vi "DetectDev.vi"(1 "IP.":string caption="IP地址") -> (0 "Fail":bool)   [LabVIEW 2012]
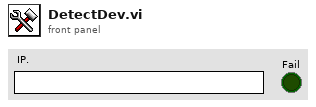
[diagram p1: front panel]
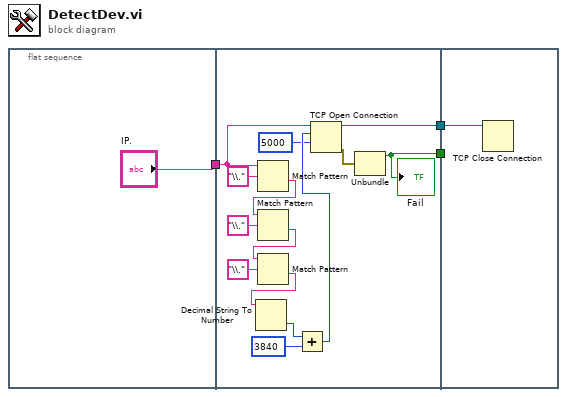
[diagram p0: block diagram]
diagram:
  n1 = flat-sequence {
    tunnel: ["IP."] -> w3
    tunnel: w3 -> [w13]
    tunnel: [w7] -> w2
    tunnel: [w6] -> w1
    tunnel: w2 -> [w19]
    tunnel: w1 -> [_]
    frame #0 {
    }
    frame #1 {
      n2 = Match Pattern(string=w13, regular expression="\\." ("正则表达式")) -> (after substring=w15:string)  [unwired: 1 in, 3 out]
      n3 = Match Pattern(string=w15, regular expression="\\." ("正则表达式")) -> (after substring=w14:string)  [unwired: 1 in, 3 out]
      n4 = Match Pattern(string=w14, regular expression="\\." ("正则表达式")) -> (after substring=w12:string)  [unwired: 1 in, 3 out]
      n5 = Decimal String To Number(string=w12) -> (number=w11:i32)  [unwired: 2 in, 1 out]
      n6 = Add(x=w11, y=3840) -> (x+y=w9:i32)
      n7 = TCP Open Connection(address=w13, remote port or service name=w9, timeout ms (60000)=5000 ("超时毫秒(60000)")) -> (connection ID=w7:refnum<k5>, error out=w8:errorcluster)  [unwired: 2 in]
      n8 = Unbundle(w8) -> ("status"=w6:bool)  [unwired: 2 out]
      "Fail" <- w6
    }
    frame #2 {
      n9 = TCP Close Connection(connection ID=w19) -> ()  [unwired: 2 in, 2 out]
    }
  }
